vi "Tick.vi"(11 "Actor in":refnum<class "Actor.lvclass">) -> ()   [LabVIEW 2020, in "Actor.lvclass"]
uses:
  Actor.lvclass
  Sequencer/Sequencer.lvclass
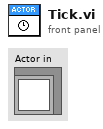
[diagram p1: front panel]
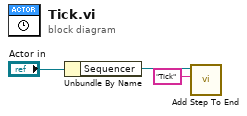
[diagram p0: block diagram]
diagram:
  n1 = Unbundle By Name("Actor in") -> ("Sequencer"=w2:refnum<class "Sequencer.lvclass">)
  n2 = call "Add Step To End.vi"("Step Name"="Tick", "Sequencer in"=w2) -> ()  [unwired: 9 in, 1 out]
